vi "SearchMATArrayForPos.vi"(3 "pixel per line":i32, 4 "macro times":dbl[](array[numeric])) -> (1 "Array":i32[](array[numeric]))   [LabVIEW 2009]
uses:
  <vilib>/Analysis/NI_AALPro.lvlib
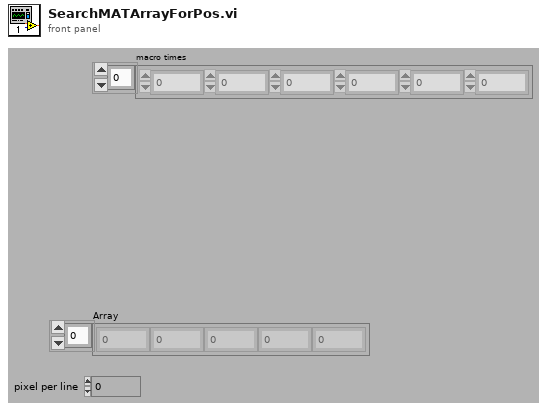
[diagram p1: front panel]
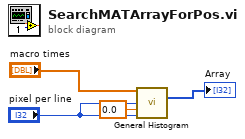
[diagram p0: block diagram]
diagram:
  n1 = call <vilib>:"General Histogram.vi"("X"="macro times", "max"="pixel per line", "min"=0.0, "# bins"="pixel per line") -> ("Histogram"=→"Array":i32[])  [unwired: 7 in, 4 out]
